vi "Test Client.vi"() -> ()   [LabVIEW 2016, in "Instrument.SR7270.lvclass"]
uses:
  Instrument.SR7270.lvclass
  levylab_util_remote/src/SMOs/RemoteControl/Typedefs/Message--Cluster.ctl
  <userlib>/_OpenG.lib/numeric/numeric.llb/Random Number Within Range - DBL__ogtk.vi
  levylab_util_remote/src/SMOs/RemoteControl/RemoteControl.lvclass
panel:
  out "Numeric":i32
  in  "stop":bool
  out "Waveform Chart":u32(graph)
  out "error out":errorcluster
  out "execution time (ms)":u32
  out "Message Received":T1
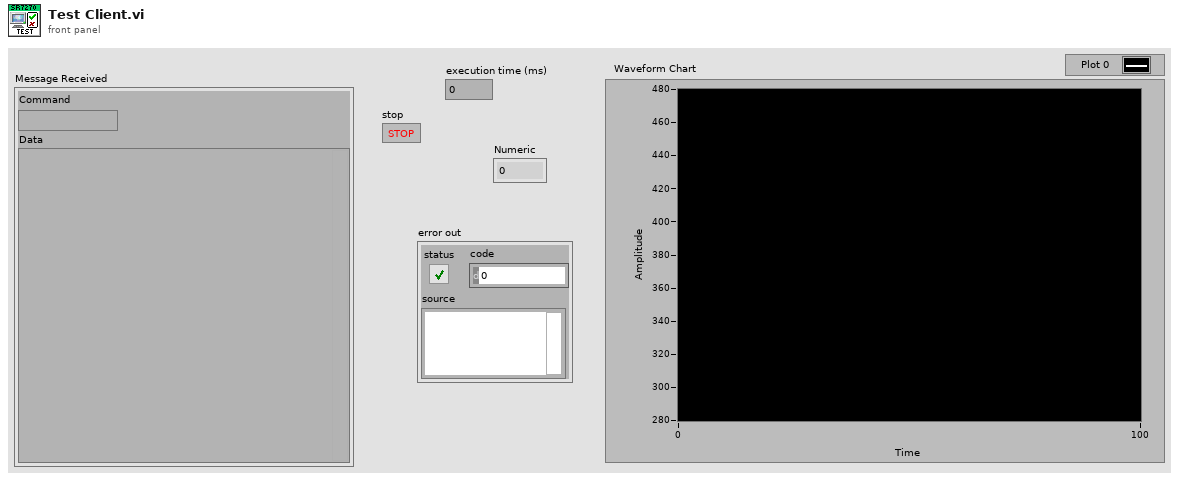
[diagram p1: front panel]
types:
  T1 = typedef "RemoteControl.lvclass/Message--Cluster.ctl" = cluster{"Command":string, "Data":variant}
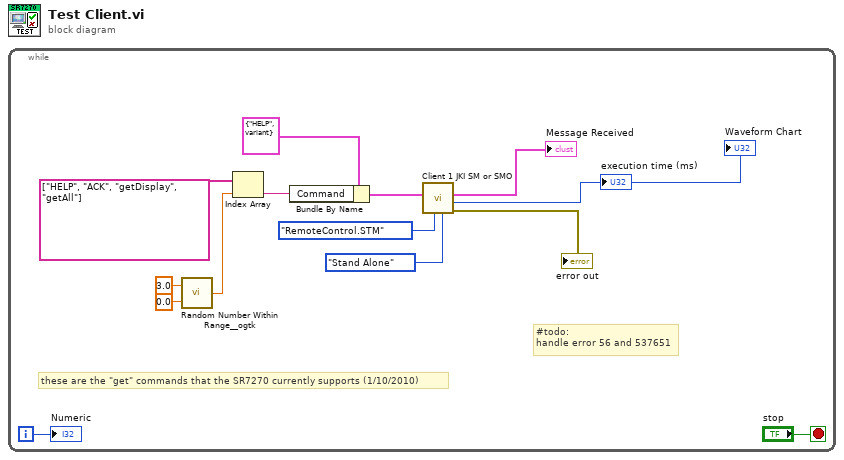
[diagram p0: block diagram]
diagram:
  n1 = while {
    i -> [w3]
    stop <- "stop" stop-if-true
    # "#todo:\nhandle error 56 and 537651"
    # "these are the \"get\" commands that the SR7270 currently supports (1/10/2010)"
    n2 = call-poly <userlib>:"Random Number Within Range__ogtk.vi"("High"=3.0, "Low"=0.0) -> ("Random Number"=w8:dbl)  [unwired: 3 in]
    n3 = Index Array(array=string[] ["HELP", "ACK", "getDisplay", "getAll"], index=w8) -> (element=w11:string)
    n4 = Bundle By Name(cluster=T1 {"Command"="HELP", "Data"=variant} ("Message to Send"), "Command"=w11) -> (w13:T1)
    n5 = call "Client 1 JKI SM or SMO.vi"("Enum 2"=enum16{"SMO", "Stand Alone"}."Stand Alone", "Enum"=enum16{"RemoteControl", "RemoteControl.STM"}."RemoteControl.STM", "Message to Send"=w13) -> ("error out"=→"error out":errorcluster, "execution time (ms)"=→"execution time (ms)" →"Waveform Chart":u32, "Message Received"=→"Message Received":T1)  [unwired: 6 in]
    "Numeric" <- w3
  }
